vi "获取当前时间-秒.vi"() -> (3 "秒":dbl)   [LabVIEW 2013]
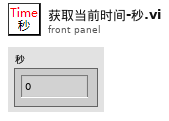
[diagram p1: front panel]
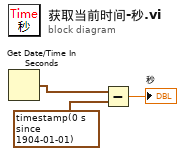
[diagram p0: block diagram]
diagram:
  n1 = Get Date/Time In Seconds() -> (seconds since 1Jan1904=w1:timestamp)
  n2 = Subtract(x=w1, y=timestamp(0 s since 1904-01-01)) -> (x-y=→"秒":dbl)
